vi "属性节点和枚举.vi"() -> ()   [LabVIEW 2018]
panel:
  out "字符串":string
  out "结果":dbl caption="no"
  in  "枚举":enum16{"12", "15", "18", ""}(ring)
  # "这里是标题而非标签"
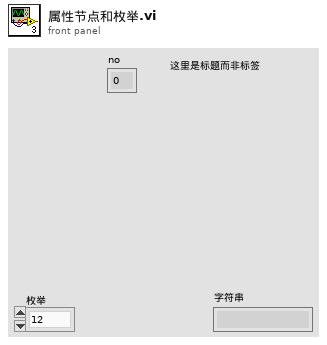
[diagram p1: front panel]
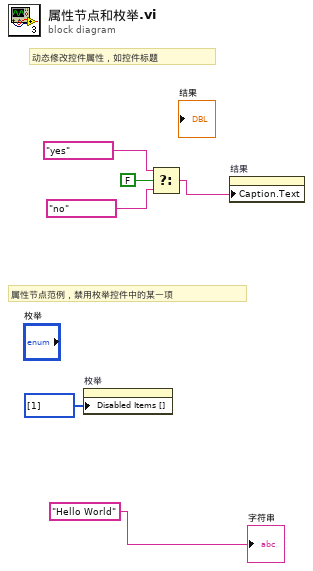
[diagram p0: block diagram]
diagram:
  # "动态修改控件属性，如控件标题"
  # "属性节点范例，禁用枚举控件中的某一项"
  n1 = property on="枚举" class="Enum (严格)"("Disabled Items []"=i32[] [1] ("禁用项[]")) -> ()  [unwired: 2 in, 2 out]
  n2 = Select(t="yes", s=FALSE, f="no") -> (s? t:f=w5:string)
  n3 = property on="结果" class="DigNum (严格)"("Caption.Text"=w5) -> ()  [unwired: 2 in, 2 out]
  "字符串" <- "Hello World"
